vi "SaveDatabase (SubVI).vi"(3 "error in (no error)":errorcluster, 4 "Datos":T1={"Imei"="359772033694416", "Evento"="Automático", "Lat"="-2.884192", "Lon"="-79.012285", "F_H_eve"=timestamp(3439900564 s since 1904-01-01), "F_H_rec"=timestamp(3447157248.23 s since 1904-01-01)}, 5 "Refnum in":T2) -> (0 "error out":errorcluster, 2 "Refnum out":T2)   [LabVIEW 2012]
uses:
  <vilib>/addons/database/Connection.llb/Conn ObjectReference.ctl
  <vilib>/addons/database/Auxilliary.llb/DB Tools Parameter Info.ctl
  <vilib>/addons/database/Auxilliary.llb/DB Tools DataTypes.ctl
  <vilib>/addons/database/Auxilliary.llb/DB Tools Parameter Dir.ctl
  <vilib>/addons/database/Auxilliary.llb/DB Tools Format Datetime String (Time Stamp).vi
  <vilib>/addons/database/Command.llb/Cmd Set Parameter Value (C).vi
  <vilib>/addons/database/Command.llb/Cmd Execute.vi
  <vilib>/addons/database/Recordset.llb/Rec Destroy - Command.vi
  <vilib>/addons/database/Command.llb/Cmd Delete.vi
  <vilib>/addons/database/NI_Database_API.lvlib
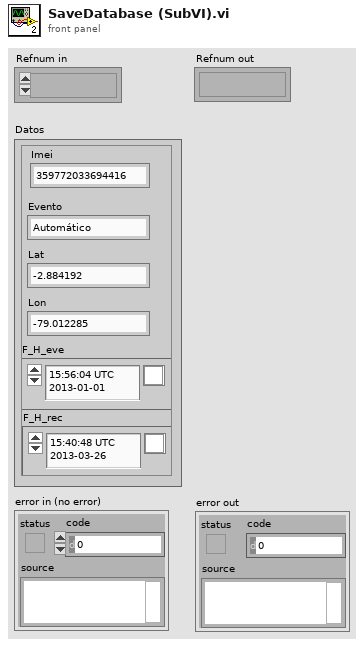
[diagram p1: front panel]
types:
  T1 = cluster{"Imei":string, "Evento":string, "Lat":string, "Lon":string, "F_H_eve":timestamp, "F_H_rec":timestamp}
  T2 = typedef "NI_Database_API.lvlib/Conn ObjectReference.ctl" = refnum<k1>
  T3 = typedef "NI_Database_API.lvlib/DB Tools Parameter Info.ctl" = cluster{"parameter name":string, "type":T4, "direction":T5, "value":variant}
  T4 = typedef "NI_Database_API.lvlib/DB Tools DataTypes.ctl" = enum16{"String", "Long (I32)", "Single (SGL)", "Double (DBL)", "Date/Time", "Binary"}
  T5 = typedef "NI_Database_API.lvlib/DB Tools Parameter Dir.ctl" = enum32{"Input", "Output", "Input/Output", "Return Value"}
  T6 = typedef "NI_Database_API.lvlib/Cmd ObjectReference.ctl" = refnum<k1>
  T7 = typedef "NI_Database_API.lvlib/Cmd-Rec Object Reference.ctl" = refnum<k1>
  T8 = cluster{"Evento":string, "Lat":string, "Lon":string, "F_H_eve":timestamp, "F_H_rec":timestamp}
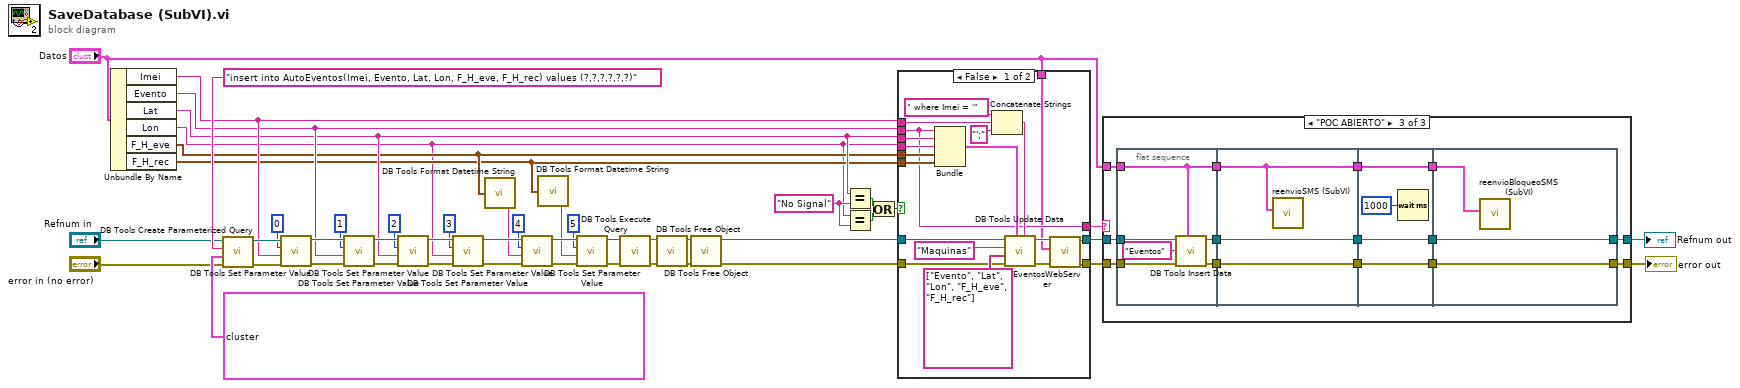
[diagram p0: block diagram]
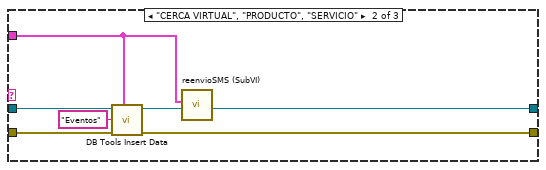
[diagram p3: hidden frame]
diagram:
  w45 = "No Signal" ("y")
  n1 = Unbundle By Name("Datos") -> ("Imei"=w26:string, "Evento"=w25:string, "Lat"=w24:string, "Lon"=w9:string, "F_H_eve"=w12:timestamp, "F_H_rec"=w10:timestamp)
  n2 = call <vilib>:"DB Tools Create Parameterized Query.vi"("error in (no error)"="error in (no error)", "parameters"=T3[] [{"parameter name"="Imei", "type"=enum."String", "direction"=enum."Input", "value"=variant}, {"parameter name"="Evento", "type"=enum."String", "direction"=enum."Input", "value"=variant}, {"parameter name"="Lat", "type"=enum."String", "direction"=enum."Input", "value"=variant}, {"parameter name"="Lon", "type"=enum."String", "direction"=enum."Input", "value"=variant}, {"parameter name"="F_H_eve", "type"=enum."Date/Time", "direction"=enum."Input", "value"=variant}, {"parameter name"="F_H_rec", "type"=enum."Date/Time", "direction"=enum."Input", "value"=variant}], "SQL query"="insert into AutoEventos(Imei, Evento, Lat, Lon, F_H_eve, F_H_rec) values (?,?,?,?,?,?)", "connection reference"="Refnum in") -> ("error out"=w30:errorcluster, "command reference"=w29:T6)  [unwired: 3 in, 1 out]
  n3 = call-poly <vilib>:"DB Tools Set Parameter Value.vi"("error in (no error)"=w30, "value"=w26, "parameter index"=0, "command reference"=w29) -> ("error out"=w42:errorcluster, "command reference out"=w41:T6)  [unwired: 4 in]
  n4 = call-poly <vilib>:"DB Tools Set Parameter Value.vi"("error in (no error)"=w42, "value"=w25, "parameter index"=1, "command reference"=w41) -> ("error out"=w40:errorcluster, "command reference out"=w39:T6)  [unwired: 4 in]
  n5 = call-poly <vilib>:"DB Tools Set Parameter Value.vi"("error in (no error)"=w40, "value"=w24, "parameter index"=2, "command reference"=w39) -> ("error out"=w32:errorcluster, "command reference out"=w31:T6)  [unwired: 4 in]
  n6 = call-poly <vilib>:"DB Tools Set Parameter Value.vi"("error in (no error)"=w32, "value"=w9, "parameter index"=3, "command reference"=w31) -> ("error out"=w33:errorcluster, "command reference out"=w34:T6)  [unwired: 4 in]
  n7 = call-poly <vilib>:"DB Tools Format Datetime String.vi"("time stamp"=w12) -> ("date/time string"=w13:string)
  n8 = call-poly <vilib>:"DB Tools Set Parameter Value.vi"("error in (no error)"=w33, "value"=w13, "parameter index"=4, "command reference"=w34) -> ("error out"=w22:errorcluster, "command reference out"=w23:T6)  [unwired: 4 in]
  n9 = call-poly <vilib>:"DB Tools Format Datetime String.vi"("time stamp"=w10) -> ("date/time string"=w11:string)
  n10 = call-poly <vilib>:"DB Tools Set Parameter Value.vi"("error in (no error)"=w22, "value"=w11, "parameter index"=5, "command reference"=w23) -> ("error out"=w20:errorcluster, "command reference out"=w21:T6)  [unwired: 4 in]
  n11 = call-poly <vilib>:"DB Tools Execute Query.vi"("error in (no error)"=w20, "command reference"=w21) -> ("error out"=w38:errorcluster, "command-recordset reference"=w37:T7)  [unwired: 6 in]
  n12 = call-poly <vilib>:"DB Tools Free Object.vi"("error in (no error)"=w38, "command-recordset reference"=w37) -> ("error out"=w35:errorcluster, "command reference"=w36:T6)  [unwired: 8 in]
  n13 = call-poly <vilib>:"DB Tools Free Object.vi"("error in (no error)"=w35, "command reference"=w36) -> ("error out"=w27:errorcluster, "connection reference"=w28:T2)  [unwired: 8 in]
  n14 = Equal?(x=w24, y=w45) -> (x = y?=w47:bool)
  n15 = Equal?(x=w9, y=w45) -> (x = y?=w48:bool)
  n16 = Or(x=w47, y=w48) -> (x .or. y?=w46:bool)
  n17 = case shown="False" w46 {
    tunnel: [w50 w70] -> w5
    tunnel: [w52 w69] -> w6
    tunnel: w10 -> [w61 _]
    tunnel: w12 -> [w60 _]
    tunnel: w9 -> [w59 _]
    tunnel: w24 -> [w58 _]
    tunnel: w25 -> [w54 w68]
    tunnel: w26 -> [w57 _]
    tunnel: w28 -> [w56 w70]
    tunnel: w27 -> [w55 w69]
    tunnel: [w54 w68] -> w2
    tunnel: "Datos" -> [w49 _]
    frame False {
      n18 = Bundle("Evento"=w54, "Lat"=w58, "Lon"=w59, "F_H_eve"=w60, "F_H_rec"=w61) -> (w62:T8)  [unwired: 1 in]
      n19 = Concatenate Strings(" where Imei = '" ("Substring"), w57, "';") -> (w65:string)
      n20 = call <vilib>:"DB Tools Update Data.vi"("condition"=w65, "data"=w62, "error in (no error)"=w55, "columns"=string[] ["Evento", "Lat", "Lon", "F_H_eve", "F_H_rec"], "table"="Maquinas", "connection reference"=w56) -> ("error out"=w53:errorcluster, "connection reference out"=w51:T2)  [unwired: 4 in]
      n21 = call "EventosWebServer.vi"("error in (no error)"=w53, "Datos"=w49, "Refnum in"=w51) -> ("error out"=w52:errorcluster, "Refnum out"=w50:T2)  [unwired: 7 in]
    }
    frame True {
    }
  }
  n22 = case shown="\"POC ABIERTO\"" w2 {
    tunnel: w6 -> [w71 w77 w92]
    tunnel: w5 -> [w72 w76 w91]
    tunnel: [w72 w75 w90] -> w4
    tunnel: [w71 w74 w89] -> w3
    tunnel: "Datos" -> [_ w73 w88]
    frame Default {
    }
    frame "CERCA VIRTUAL", "PRODUCTO", "SERVICIO" {
      n23 = call <vilib>:"DB Tools Insert Data.vi"("data"=w73, "error in (no error)"=w77, "table"="Eventos", "connection reference"=w76) -> ("error out"=w74:errorcluster, "connection reference out"=w75:T2)  [unwired: 6 in]
      n24 = call "reenvioSMS (SubVI).vi"("Datos"=w73) -> ()  [unwired: 11 in]
    }
    frame "POC ABIERTO" {
      n25 = flat-sequence {
        tunnel: w92 -> [w97]
        tunnel: w91 -> [w96]
        tunnel: w88 -> [w93]
        tunnel: [w95] -> w87
        tunnel: [w94] -> w86
        tunnel: [w93] -> w85
        tunnel: w87 -> [w101]
        tunnel: w86 -> [w100]
        tunnel: w85 -> [w99]
        tunnel: [w101] -> w84
        tunnel: [w100] -> w82
        tunnel: [w99] -> w80
        tunnel: w84 -> [w105]
        tunnel: [w105] -> w83
        tunnel: w82 -> [w104]
        tunnel: [w104] -> w81
        tunnel: w80 -> [w103]
        tunnel: [w103] -> w79
        tunnel: [w107] -> w89
        tunnel: [w108] -> w90
        tunnel: w83 -> [w108]
        tunnel: w81 -> [w107]
        tunnel: w79 -> [w106]
        frame #0 {
          n26 = call <vilib>:"DB Tools Insert Data.vi"("data"=w93, "error in (no error)"=w97, "table"="Eventos", "connection reference"=w96) -> ("error out"=w94:errorcluster, "connection reference out"=w95:T2)  [unwired: 6 in]
        }
        frame #1 {
          n27 = call "reenvioSMS (SubVI).vi"("Datos"=w99) -> ()  [unwired: 11 in]
        }
        frame #2 {
          n28 = Wait (ms)(milliseconds to wait=u32 1000) -> ()  [unwired: 1 out]
        }
        frame #3 {
          n29 = call "reenvioBloqueoSMS (SubVI).vi"("Datos"=w106) -> ()  [unwired: 11 in]
        }
      }
    }
  }
  "error out" <- w3
  "Refnum out" <- w4
